vi "Load Plugin Timeout.vi"(8 "error in (no error)":errorcluster, 10 "New Plugin":T1, 11 "CIFPluginManager in":refnum<class "CIFPluginManager.lvclass">) -> (0 "error out":errorcluster)   [LabVIEW 2021, in "CIFPluginManager.lvclass"]
uses:
  CIFPluginManager.lvclass
  CIFPluginManager.lvclass/CIFPluginManager.ctl
  CIFCore/Common/Typedef/Errors.ctl
  CIFCore/Common/CIFCoreCommon.lvlib
  typedef/Loader Type.ctl
  typedef/Plugin Load Command.ctl
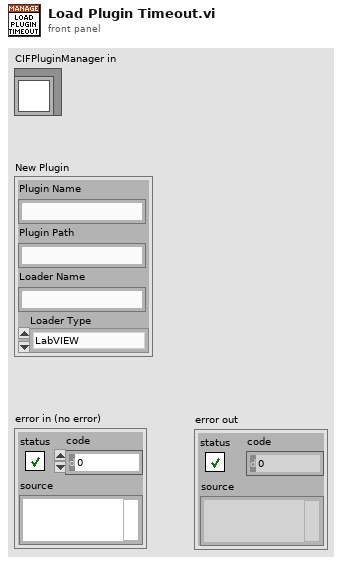
[diagram p1: front panel]
types:
  T1 = typedef "CIFPluginManager.lvclass/Plugin Load Command.ctl" = cluster{"Plugin Name":string, "Plugin Path":string, "Loader Name":string, "Loader Type":T2}
  T2 = typedef "CIFPluginManager.lvclass/Loader Type.ctl" = enum16{"LabVIEW"}
  T3 = typedef "CIFCoreCommon.lvlib/Errors.ctl" = enum16{"Invalid Clock ID", "Long Sleep", "gRPC Server Not Found", "Config Parse", "Timestamp Wrap", "Delayed Execution", "Duplicate Channel", "Missing Channel", "Incorrect Type", "Flatten Error", "Unflatten Data", "Unique Name", "Plugin Not Found", "Plugin Type Not Found", "Plugin Version Not Found", "Manager Not Found", "Numerical Issue", "Time Jump", "Clock ID Match", "Channel Length", "Plugin Connection", "gRPC Server Connection", "PPL Name Match", "Build", "Config Log Parse", "Plugin Load", "UI Subpanel Load", "Python Name", "Invalid Name", "Unable to Change Ch Buffer", "Failed Kill", "Failed SysExec", "Function Not Implemented", "Load Timeout"}
  T4 = typedef "CIFPluginManager.lvclass/Plugin Management Data Map.ctl" = map{string, T5}
  T5 = typedef "CIFPluginManager.lvclass/Plugin Management Data.ctl" = cluster{"Unique Name":string, "Plugin Type":string, "gRPC Port":i32, "gRPC ID":T6, "Loader Type":T2, "Loader":string, "Version":T7, "Load Timestamp":i64, "Unload Timestamp":i64, "Unloading":bool, "Ready for removal":bool, "status":T8, "channels":T17}
  T6 = typedef "grpc-lvsupport-release.lvlib/grpcId.ctl" = u64
  T7 = typedef "CIFCoreCommon.lvlib/Version.ctl" = cluster{"Major":i32, "Minor":i32, "Fix":i32, "Build":i32}
  T8 = typedef "CIF_Manager_server.lvlib/cif_plugincore_StatusData.ctl" = cluster{"state":T9, "timing_statistics":T10, "fifo_statistics":T12, "error":T13, "monitor_doubles":T14, "monitor_u64s":T15, "monitor_i64s":T16}
  T9 = typedef "CIF_Manager_server.lvlib/cif_plugincore_StatusData_PluginState.ctl" = enum32{"PLUGINSTATE_UNKNOWN", "PLUGINSTATE_CREATING", "PLUGINSTATE_LISTENING", "PLUGINSTATE_RUNNING", "PLUGINSTATE_CLEANINGUP", "PLUGINSTATE_DESTROYING"}
  T10 = typedef "CIF_Manager_server.lvlib/cif_plugincore_TimingStatistics.ctl" = cluster{"period":T11, "wake_error":T11, "execute":T11, "housekeep":T11, "idle":T11, "cleanup":T11, "custom_1":T11, "custom_2":T11}
  T11 = typedef "CIF_Manager_server.lvlib/cif_common_TimingStats.ctl" = cluster{"max":i64, "min":i64, "avg":dbl}
  T12 = typedef "CIF_Manager_server.lvlib/cif_plugincore_FifoStatistics.ctl" = cluster{"from_t0":T11, "from_previous_plugin":T11, "output_error":T11}
  T13 = typedef "CIF_Manager_server.lvlib/cif_plugincore_Error.ctl" = cluster{"status":bool, "code":i32}
  T14 = typedef "CIF_Manager_server.lvlib/cif_plugincore_MonitorDoubles.ctl" = cluster{"double_1":dbl, "double_2":dbl, "double_3":dbl, "double_4":dbl}
  T15 = typedef "CIF_Manager_server.lvlib/cif_plugincore_MonitorU64.ctl" = cluster{"u64_1":u64, "u64_2":u64, "u64_3":u64, "u64_4":u64}
  T16 = typedef "CIF_Manager_server.lvlib/cif_plugincore_MonitorI64.ctl" = cluster{"i64_1":i64, "i64_2":i64, "i64_3":i64, "i64_4":i64}
  T17 = typedef "CIF_Manager_server.lvlib/cif_channelcore_Channels.ctl" = cluster{"channels":T18[]}
  T18 = typedef "CIF_Manager_server.lvlib/cif_channelcore_Channel.ctl" = cluster{"name":string, "direction":T19, "type":string, "custom_config":u8[], "connected":bool, "connected_name":string, "forced":bool, "channel_pattern":T20}
  T19 = typedef "CIF_Manager_server.lvlib/cif_channelcore_ChannelDirection.ctl" = enum32{"CHANNELDIRECTION_UNKNOWN", "CHANNELDIRECTION_PUBLISHER", "CHANNELDIRECTION_SUBSCRIBER"}
  T20 = typedef "CIF_Manager_server.lvlib/cif_channelcore_ChannelPattern.ctl" = enum32{"CHANNELPATTERN_UNKNOWN", "CHANNELPATTERN_TAG", "CHANNELPATTERN_FIFO", "CHANNELPATTERN_MULTIFIFO", "CHANNELPATTERN_BACKPRESSUREFIFO"}
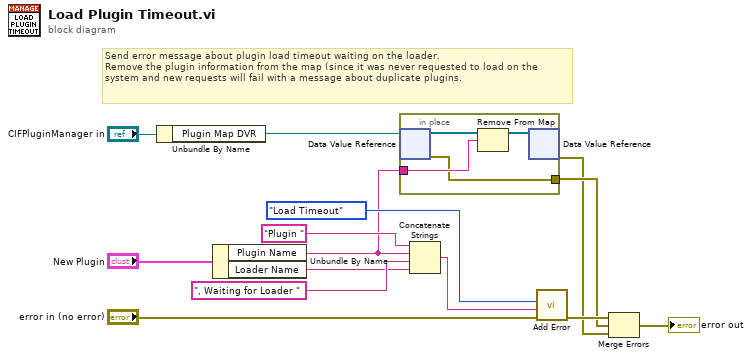
[diagram p0: block diagram]
diagram:
  # "Send error message about plugin load timeout waiting on the loader.\nRemove the plugin information from the map (since it was never requested to load on the system and new requests will fail with a message about duplicate plugins."
  n1 = Unbundle By Name("CIFPluginManager in") -> ("Plugin Map DVR"=w6:refnum<data-value>)
  n2 = Unbundle By Name("New Plugin") -> ("Plugin Name"=w5:string, "Loader Name"=w8:string)
  n3 = in-place {
    in-place-border: w5 -> [w16]
    in-place-border: [w15] -> w3
    n4 = in-place-dvr #1(w6) -> (w18:T4, w15:errorcluster)
    n5 = Remove From Map(10:w16, 11:w18) -> (3:w17:T4)  [unwired: 2 out]
    n6 = in-place-dvr #1(w17) -> (w2:errorcluster)  [unwired: 1 out]
  }
  n7 = Concatenate Strings("Plugin " ("String to Append"), w5, ", Waiting for Loader " ("string"), w8) -> (w10:string)
  n8 = call "Add Error.vi"("error in (no error)"="error in (no error)", "String to Append"=w10, "Error"=Errors."Load Timeout") -> ("error out"=w4:errorcluster)  [unwired: 8 in]
  n9 = Merge Errors(w4, w3, w2) -> (→"error out":errorcluster)
